vi "TEST.vi"() -> ()   [LabVIEW 2016, in "ENED1100-UCBA-Sensor-Motor-Testing.lvrbt"]
uses:
  ENED1100-UCBA-Sensor-Motor-Testing.lvrbt
  <vilib>/NXT/Subs/LVHSConnector.ctl
  <vilib>/NXT/LegoClasses/BrickReference/BrickReference.lvclass
  <vilib>/NXT/Block Support/NXT_OutputPort.ctl
  <vilib>/NXT/NXTIO Xnodes/NXTIONodeSubVIs/LEGOMotorStatus.vi
  <vilib>/NXT/NXTIO Xnodes/NXTIONodeSubVIs/NXTMotorRunDistance.vi
  <vilib>/NXT/NXTIO Xnodes/NXTIONodeSubVIs/NXTStopMotors.vi
  <vilib>/NXT/NXTIO Xnodes/AddressXNode/NXTIOAddress.xnode
  <vilib>/NXT/NXTIO Xnodes/NXTIOXNode/NXTIO.xnode
panel:
  out "Moving 1":bool
  in  "NXT/EV3":T1
  out "NXT/EV3 2":T1
  in  "Speed 1":i8=75
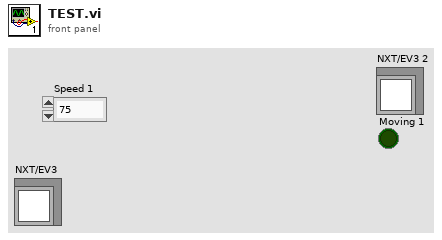
[diagram p1: front panel]
types:
  T1 = typedef "LVHSConnector.ctl" = refnum<class "BrickReference.lvclass">
  T2 = typedef "NXT_OutputPort.ctl" = u8
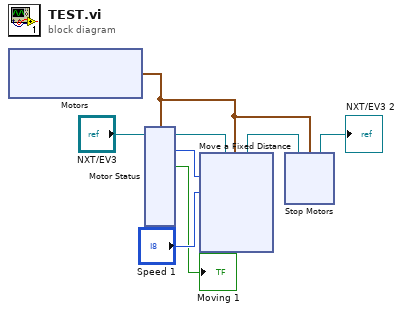
[diagram p0: block diagram]
diagram:
  n1 = xnode "Motors"() -> ("Motor"=w1:cluster{"Port":T2, "Port":T2})
  n2 = xnode "Motor Status"("Motors"=w1, "NXT/EV3"="NXT/EV3") -> ("Moving 1"=→"Moving 1":bool, "Position 1"=w2:i32, "NXT/EV3"=w5:T1)  [unwired: 2 out]
  n3 = xnode "Move a Fixed Distance"("Speed 1"="Speed 1", "Distance 1"=w2, "Motors"=w1, "NXT/EV3"=w5) -> ("NXT/EV3"=w7:T1)  [unwired: 2 in]
  n4 = xnode "Stop Motors"("Motors"=w1, "NXT/EV3"=w7) -> ("NXT/EV3"=→"NXT/EV3 2":T1)
